vi "Keithley2450 DC Pulses Blocks with Ramps.vi"(4 "Compliance(V)":dbl=210.0, 5 "VISA resource name":refnum<visa-resource-name>, 6 "Source Mode":enum16{"Voltage", "Current"}(ring)=enum."Current", 7 "Full Ramp\nTime (sec)":dbl, 8 "Second Pulse\nTime (sec)":dbl, 9 "Second Pulse\nAmplitude (mU)":dbl, 10 "First Pulse\nTime (sec)":dbl, 11 "First Pulse\nAmplitude (mU)":dbl) -> (0 "Remaining\nTime (s)":dbl format="%<%M:%S%1u>t", 1 "Total Time (s)":dbl, 2 "Charge (mC)":dbl, 3 "Output Waveform":waveform(dbl)(graph))   [LabVIEW 2020]
uses:
  <vilib>/Analysis/1siggen.llb/Ramp Pattern by Samples.vi
  <vilib>/Waveform/WDTOps.llb/WDT Append Waveforms DBL.vi
  <instrlib>/Keithley 2450/Public/Data/Read (Multiple Points).vi
  <vilib>/measure/NI_MAPro.lvlib
  <vilib>/Analysis/NI_AALBase.lvlib
  <instrlib>/Keithley 2450/Keithley 2450.lvlib
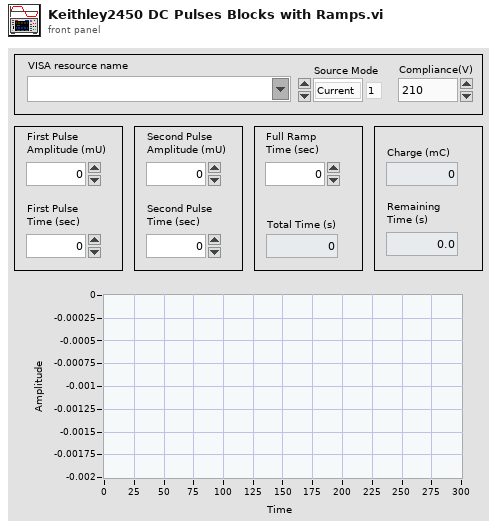
[diagram p1: front panel]
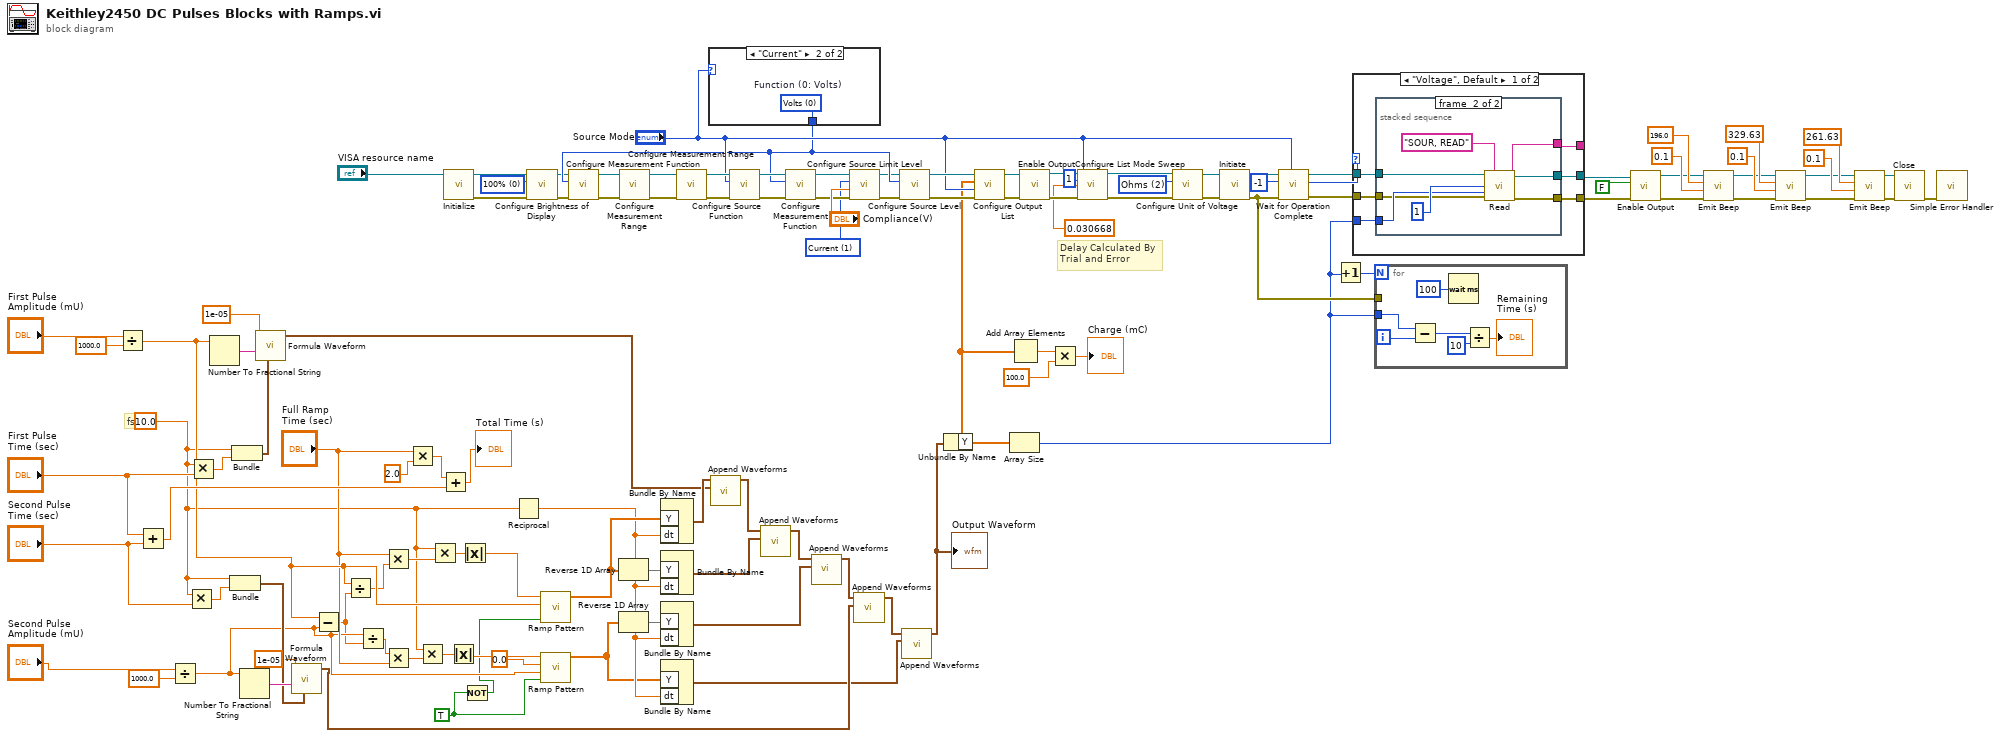
[diagram p0: block diagram]
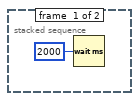
[diagram p2: hidden frame]
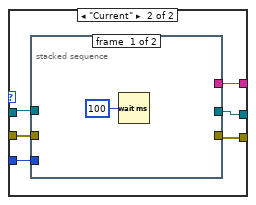
[diagram p3: hidden frame]
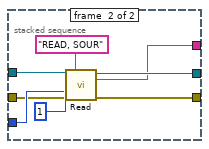
[diagram p4: hidden frame]
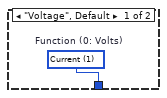
[diagram p5: hidden frame]
diagram:
  w1 = u16 0 items=["100%", "75%", "50%", "25%", "Display Off", "Display and Indicators Off"] ("Brightness (0: 100%)")
  w26 = u16 2 items=["Volts", "Watts", "Ohms"] ("Unit (0: Volts)")
  w40 = TRUE ("exclude end?")
  w82 = u16 1 items=["Volts", "Current"] ("Function (0: Volts)")
  w64 = 10.0
  # "Delay Calculated By\nTrial and Error"
  # "fs"
  n1 = Divide(x="First Pulse\nAmplitude (mU)", y=1000.0) -> (x/y=w69:dbl)
  n2 = Add(x="First Pulse\nTime (sec)", y="Second Pulse\nTime (sec)") -> (x+y=w73:dbl)
  n3 = Divide(x="Second Pulse\nAmplitude (mU)", y=1000.0) -> (x/y=w62:dbl)
  n4 = Multiply(x=w64, y="Second Pulse\nTime (sec)") -> (x*y=w113:dbl)
  n5 = Multiply(x=w64, y="First Pulse\nTime (sec)") -> (x*y=w114:dbl)
  n6 = Number To Fractional String(number=w69) -> (F-format string=w112:string)  [unwired: 3 in]
  n7 = Bundle(w64, w113) -> (w109:cluster{dbl, dbl})  [unwired: 1 in]
  n8 = Bundle(w64, w114) -> (w111:cluster{dbl, dbl})  [unwired: 1 in]
  n9 = Number To Fractional String(number=w62) -> (F-format string=w110:string)  [unwired: 3 in]
  n10 = call <vilib>:"Formula Waveform.vi"("sampling info"=w111, "formula"=w112, "frequency"=1e-05) -> ("signal out"=w60:waveform(dbl))  [unwired: 7 in, 1 out]
  n11 = call <vilib>:"Formula Waveform.vi"("sampling info"=w109, "formula"=w110, "frequency"=1e-05) -> ("signal out"=w51:waveform(dbl))  [unwired: 7 in, 1 out]
  n12 = Subtract(x=w69, y=w62) -> (x-y=w46:dbl)
  n13 = Divide(x=w69, y=w46) -> (x/y=w68:dbl)
  n14 = Divide(x=w62, y=w46) -> (x/y=w65:dbl)
  n15 = Multiply(x="Full Ramp\nTime (sec)", y=w68) -> (x*y=w67:dbl)
  n16 = Multiply(x=w65, y="Full Ramp\nTime (sec)") -> (x*y=w63:dbl)
  n17 = Multiply(x="Full Ramp\nTime (sec)", y=2.0) -> (x*y=w72:dbl)
  n18 = Multiply(x=w64, y=w63) -> (x*y=w43:dbl)
  n19 = Multiply(x=w64, y=w67) -> (x*y=w45:dbl)
  n20 = Add(x=w72, y=w73) -> (x+y=→"Total Time (s)":dbl)
  n21 = call <instrlib>:"Initialize.vi"("VISA resource name"="VISA resource name") -> ("error out"=w3:errorcluster, "VISA resource name out"=w2:refnum<visa-resource-name>)  [unwired: 9 in]
  n22 = Absolute Value(x=w43) -> (abs(x)=w42:dbl)
  n23 = Absolute Value(x=w45) -> (abs(x)=w44:dbl)
  n24 = Not(x=w40) -> (.not. x?=w39:bool)
  n25 = Reciprocal(x=w64) -> (1/x=w56:dbl)
  n26 = call <instrlib>:"Configure Brightness of Display.vi"("error in (no error)"=w3, "Brightness (0: 100%)"=w1, "VISA resource name"=w2) -> ("error out"=w4:errorcluster, "VISA resource name out"=w5:refnum<visa-resource-name>)  [unwired: 7 in]
  n27 = call-poly <vilib>:"Ramp Pattern.vi"("exclude end?"=w39, "end"=w69, "samples"=w44) -> ("Ramp Pattern"=w57:dbl[])  [unwired: 7 in, 1 out]
  n28 = call-poly <vilib>:"Ramp Pattern.vi"("exclude end?"=w40, "start"=w62, "end"=0.0, "samples"=w42) -> ("Ramp Pattern"=w48:dbl[])  [unwired: 6 in, 1 out]
  n29 = Reverse 1D Array(array=w57) -> (reversed array=w58:dbl[])
  n30 = Reverse 1D Array(array=w48) -> (reversed array=w47:dbl[])
  n31 = Bundle By Name("Y"=w57, "dt"=w56) -> (w61:waveform(dbl))  [unwired: 1 in]
  n32 = Bundle By Name("Y"=w58, "dt"=w56) -> (w55:waveform(dbl))  [unwired: 1 in]
  n33 = Bundle By Name("Y"=w47, "dt"=w56) -> (w53:waveform(dbl))  [unwired: 1 in]
  n34 = Bundle By Name("Y"=w48, "dt"=w56) -> (w49:waveform(dbl))  [unwired: 1 in]
  n35 = case shown="\"Current\"" "Source Mode" {
    tunnel: [w115 w116] -> w83
    frame "Voltage", Default {
      w115 = u16 1 items=["Volts", "Current", "Resistance"]  # Function (0: Volts)
    }
    frame "Current" {
      w116 = u16 0 items=["Volts", "Current", "Resistance"]  # Function (0: Volts)
    }
  }
  n36 = call <instrlib>:"Configure Measurement Function.vi"("error in (no error)"=w4, "Function (0: Volts)"=w83, "VISA resource name"=w5) -> ("error out"=w99:errorcluster, "VISA resource name out"=w98:refnum<visa-resource-name>)  [unwired: 7 in]
  n37 = call <instrlib>:"Configure Measurement Range.vi"("error in (no error)"=w99, "VISA resource name"=w98) -> ("error out"=w104:errorcluster, "VISA resource name out"=w103:refnum<visa-resource-name>)  [unwired: 8 in]
  n38 = call <instrlib>:"Configure Measurement Range.vi"("error in (no error)"=w104, "VISA resource name"=w103) -> ("error out"=w97:errorcluster, "VISA resource name out"=w96:refnum<visa-resource-name>)  [unwired: 8 in]
  n39 = call-poly <vilib>:"Append Waveforms.vi"("waveform B"=w60, "waveform A"=w61) -> ("waveform out"=w59:waveform(dbl))  [unwired: 8 in, 1 out]
  n40 = call <instrlib>:"Configure Source Function.vi"("error in (no error)"=w97, "Function (0: Volts)"="Source Mode", "VISA resource name"=w96) -> ("error out"=w88:errorcluster, "VISA resource name out"=w91:refnum<visa-resource-name>)  [unwired: 7 in]
  n41 = call-poly <vilib>:"Append Waveforms.vi"("waveform B"=w55, "waveform A"=w59) -> ("waveform out"=w54:waveform(dbl))  [unwired: 8 in, 1 out]
  n42 = call <instrlib>:"Configure Measurement Function.vi"("error in (no error)"=w88, "Function (0: Volts)"=w83, "VISA resource name"=w91) -> ("error out"=w89:errorcluster, "VISA resource name out"=w90:refnum<visa-resource-name>)  [unwired: 7 in]
  n43 = call-poly <vilib>:"Append Waveforms.vi"("waveform B"=w53, "waveform A"=w54) -> ("waveform out"=w52:waveform(dbl))  [unwired: 8 in, 1 out]
  n44 = call <instrlib>:"Configure Source Limit Level.vi"("error in (no error)"=w89, "Source Limit (1.0)"="Compliance(V)", "Function (0: Volts)"=w82, "VISA resource name"=w90) -> ("error out"=w79:errorcluster, "VISA resource name out"=w80:refnum<visa-resource-name>)  [unwired: 6 in]
  n45 = call-poly <vilib>:"Append Waveforms.vi"("waveform B"=w51, "waveform A"=w52) -> ("waveform out"=w50:waveform(dbl))  [unwired: 8 in, 1 out]
  n46 = call <instrlib>:"Configure Source Level.vi"("error in (no error)"=w79, "Function (0: Volts)"=w83, "VISA resource name"=w80) -> ("error out"=w86:errorcluster, "VISA resource name out"=w87:refnum<visa-resource-name>)  [unwired: 7 in]
  n47 = call-poly <vilib>:"Append Waveforms.vi"("waveform B"=w49, "waveform A"=w50) -> ("waveform out"=w70:waveform(dbl))  [unwired: 8 in, 1 out]
  "Output Waveform" <- w70
  n48 = Unbundle By Name(w70) -> ("Y"=w33:dbl[])
  n49 = call <instrlib>:"Configure Output List.vi"("error in (no error)"=w86, "Source Mode  (0: Voltage)"="Source Mode", "Output List"=w33, "VISA resource name"=w87) -> ("error out"=w100:errorcluster, "VISA resource name out"=w101:refnum<visa-resource-name>)  [unwired: 6 in]
  n50 = Array Size(array=w33) -> (size(s)=w27:i32)
  n51 = Add Array Elements(numeric array=w33) -> (sum=w32:dbl)
  n52 = call <instrlib>:"Enable Output.vi"("error in (no error)"=w100, "VISA resource name"=w101) -> ("error out"=w95:errorcluster, "VISA resource name out"=w94:refnum<visa-resource-name>)  [unwired: 8 in]
  n53 = Multiply(x=w32, y=100.0) -> (x*y=→"Charge (mC)":dbl)
  n54 = call <instrlib>:"Configure List Mode Sweep.vi"("VISA resource name"=w94, "Source Mode  (0: Voltage)"="Source Mode", "Start Index"=u32 1, "Delay (0)"=0.030668, "error in (no error)"=w95) -> ("VISA resource name out"=w23:refnum<visa-resource-name>, "error out"=w25:errorcluster)  [unwired: 9 in]
  n55 = call <instrlib>:"Configure Unit of Voltage.vi"("error in (no error)"=w25, "Unit (0: Volts)"=w26, "VISA resource name"=w23) -> ("error out"=w24:errorcluster, "VISA resource name out"=w22:refnum<visa-resource-name>)  [unwired: 7 in]
  n56 = call <instrlib>:"Initiate.vi"("error in (no error)"=w24, "VISA resource name"=w22) -> ("error out"=w29:errorcluster, "VISA resource name out"=w34:refnum<visa-resource-name>)  [unwired: 8 in]
  n57 = call <instrlib>:"Wait for Operation Complete.vi"("error in (no error)"=w29, "Timeout (10000 ms)"=-1, "VISA resource name"=w34) -> ("error out"=w36:errorcluster, "VISA resource name out"=w35:refnum<visa-resource-name>)  [unwired: 7 in]
  n58 = Increment(x=w27) -> (x+1=w28:i32)
  n59 = case shown="\"Voltage\", Default" "Source Mode" {
    tunnel: [w122 w136] -> w81
    tunnel: [w121 w135] -> w21
    tunnel: w27 -> [w120 w137]
    tunnel: [w119 w134] -> _
    tunnel: w36 -> [w118 w133]
    tunnel: w35 -> [w117 w132]
    frame "Voltage", Default {
      n60 = stacked-sequence {
        tunnel: [_ w131] -> w122
        tunnel: [_ w130] -> w121
        tunnel: [_ w128] -> w119
        tunnel: w120 -> [_ w126]
        tunnel: w118 -> [_ w125]
        tunnel: w117 -> [_ w124]
        frame #0 {
          n61 = Wait (ms)(milliseconds to wait=u32 2000) -> ()  [unwired: 1 out]
        }
        frame #1 {
          n62 = call-poly <instrlib>:"Read.vi"("VISA resource name"=w124, "Buffer Elements"="SOUR, READ", "Start Index (1)"=1, "End Index (1)"=w126, "error in (no error)"=w125) -> ("VISA resource name out"=w131:refnum<visa-resource-name>, "Data out"=w128:string, "error out"=w130:errorcluster)  [unwired: 8 in]
        }
      }
    }
    frame "Current" {
      n63 = stacked-sequence {
        tunnel: [_ w146] -> w136
        tunnel: [_ w145] -> w135
        tunnel: [_ w143] -> w134
        tunnel: w137 -> [_ w141]
        tunnel: w133 -> [_ w140]
        tunnel: w132 -> [_ w139]
        frame #0 {
          n64 = Wait (ms)(milliseconds to wait=u32 100) -> ()  [unwired: 1 out]
        }
        frame #1 {
          n65 = call-poly <instrlib>:"Read.vi"("VISA resource name"=w139, "Buffer Elements"="READ, SOUR", "Start Index (1)"=1, "End Index (1)"=w141, "error in (no error)"=w140) -> ("VISA resource name out"=w146:refnum<visa-resource-name>, "Data out"=w143:string, "error out"=w145:errorcluster)  [unwired: 8 in]
        }
      }
    }
  }
  n66 = for {
    N: w28 -> [_]
    tunnel: w29 -> [_]
    tunnel: w27 -> [w151]
    i -> [w150]
    n67 = Subtract(x=w151, y=w150) -> (x-y=w149:i32)
    n68 = Wait (ms)(milliseconds to wait=u32 100) -> ()  [unwired: 1 out]
    n69 = Divide(x=w149, y=10) -> (x/y=→"Remaining\nTime (s)":dbl)
  }
  n70 = call <instrlib>:"Enable Output.vi"("error in (no error)"=w21, "Enable Output (T: Enable)"=FALSE, "VISA resource name"=w81) -> ("error out"=w13:errorcluster, "VISA resource name out"=w14:refnum<visa-resource-name>)  [unwired: 7 in]
  n71 = call <instrlib>:"Emit Beep.vi"("error in (no error)"=w13, "Beep Duration (.25 s)"=0.1, "Beep Frequency (300)"=196.0, "VISA resource name"=w14) -> ("error out"=w9:errorcluster, "VISA resource name out"=w10:refnum<visa-resource-name>)  [unwired: 6 in]
  n72 = call <instrlib>:"Emit Beep.vi"("error in (no error)"=w9, "Beep Duration (.25 s)"=0.1, "Beep Frequency (300)"=329.63, "VISA resource name"=w10) -> ("error out"=w8:errorcluster, "VISA resource name out"=w7:refnum<visa-resource-name>)  [unwired: 6 in]
  n73 = call <instrlib>:"Emit Beep.vi"("error in (no error)"=w8, "Beep Duration (.25 s)"=0.1, "Beep Frequency (300)"=261.63, "VISA resource name"=w7) -> ("error out"=w19:errorcluster, "VISA resource name out"=w20:refnum<visa-resource-name>)  [unwired: 6 in]
  n74 = call <instrlib>:"Close.vi"("error in (no error)"=w19, "VISA resource name"=w20) -> ("error out"=w6:errorcluster)  [unwired: 9 in]
  n75 = call <vilib>:"Simple Error Handler.vi"("error in (no error)"=w6) -> ()  [unwired: 4 in, 5 out]
